vi "Configure RemIO Module Core.vi"(8 "error in (no error)":errorcluster, 9 "module slot index":u8=1, 10 "Slave Ref In":refnum<k21>, 11 "11102 in":refnum<class "11102.lvclass">) -> (0 "error out":errorcluster, 1 "negative confirmation":u8[](array[numeric]) format="%.0x", 2 "Slave Ref Out":refnum<k21>, 3 "11102 out":refnum<class "11102.lvclass">, 5 "SDO abort code":u32 format="%.0x")   [LabVIEW 2016, in "Modules.lvlib" / "11102.lvclass"]
uses:
  11102.lvclass
  11102.lvclass/11102.ctl
  <vilib>/indcomecat/Remote IO/internal/_Configure REM-11102.vi
  <vilib>/indcomecat/Remote IO/NI ECAT Remote IO.lvlib
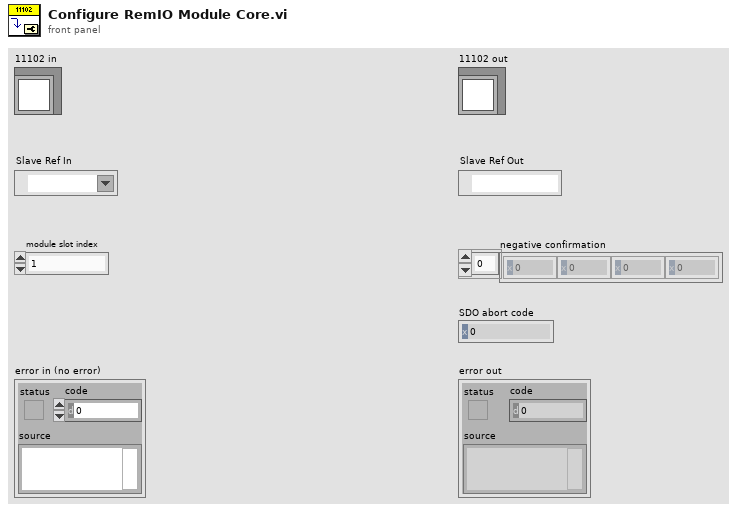
[diagram p1: front panel]
types:
  T1 = typedef "NI ECAT Remote IO.lvlib/channul number REM-11102.ctl" = u8
  T2 = typedef "NI ECAT Remote IO.lvlib/input filter time REM-11102.ctl" = u8
  T3 = typedef "NI ECAT Remote IO.lvlib/mean-value REM-11102.ctl" = u8
  T4 = typedef "NI ECAT Remote IO.lvlib/measuring range REM-11102.ctl" = u8
  T5 = cluster{"channel number":T1, "input filter time":T2, "mean-value":T3, "measuring range":T4}[]
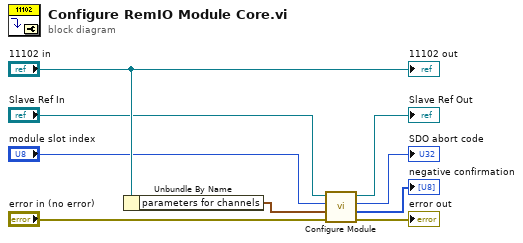
[diagram p0: block diagram]
diagram:
  n1 = Unbundle By Name("11102 in") -> ("parameters for channels"=w8:T5)
  n2 = call-poly <vilib>:"Configure Module.vi"("error in (no error)"="error in (no error)", "parameters for channels"=w8, "module slot index"="module slot index", "slave reference in"="Slave Ref In") -> ("error out"=→"error out":errorcluster, "negative confirmation"=→"negative confirmation":u8[], "SDO abort code"=→"SDO abort code":u32, "slave reference out"=→"Slave Ref Out":refnum<k21>)  [unwired: 4 in]
  "11102 out" <- "11102 in"
